vi "main(Test DQMH modules).vi"() -> ()   [LabVIEW 2018, in "Application.lvlib"] (continued)
              tunnel: w10619 -> [w10626 w10656]
              tunnel: [w10637 w10655] -> w10618
              frame False {
                w10623 = T9 {"command"="", "data"=variant} ("element")
                w10636 = T9 {"command"="", "data"=variant} ("element")
                n4774 = To Variant(anything=T3."mux10_1_channel2" ("mux10_1(x6)_encode")) -> (Variant=w10634:variant)
                n4775 = To Variant(anything=T4."demux1_10_channel2" ("demux1_10(x6)_encode")) -> (Variant=w10630:variant)
                n4776 = To Variant(anything=bool[] [FALSE, TRUE, FALSE, FALSE, FALSE, FALSE]) -> (Variant=w10645:variant)
                n4777 = Bundle By Name(cluster=w10636, "command"="MEAS.AllRelaysOFF") -> (w10644:T9)
                n4778 = Bundle By Name(cluster=w10636, "command"="MEAS.mux10-1", "data"=w10634) -> (w10627:T9)
                n4779 = Bundle By Name(cluster=w10636, "command"="MEAS.demux1-10", "data"=w10630) -> (w10628:T9)
                n4780 = Bundle By Name(cluster=w10636, "command"="MEAS.eMIC", "data"=w10645) -> (w10629:T9)
                n4781 = Build Array(w10644, w10627, w10628, w10629) -> (w10622:T9[])
                n4782 = To Variant(anything=w10626) -> (Variant=w10625:variant)
                n4783 = To Variant(anything=w10626) -> (Variant=w10624:variant)
                n4784 = Bundle By Name(cluster=w10623, "command"="MEAS.requestAC", "data"=w10625) -> (w10642:T9)
                n4785 = Bundle By Name(cluster=w10623, "command"="Apps.WaitForEvent", "data"=w10624) -> (w10638:T9)
                n4786 = Bundle By Name(cluster=w10623, "command"="Apps.UI Update 1") -> (w10639:T9)
                n4787 = Bundle By Name(cluster=w10623, "command"="WaitFor") -> (w10621:T9)
                n4788 = Build Array (concatenate)(w10622, w10621, w10642, w10638, w10639) -> (w10637:T9[])
              }
              frame True {
                w10652 = T9 {"command"="", "data"=variant} ("element")
                w10674 = T9 {"command"="", "data"=variant} ("element")
                n4789 = To Variant(anything=T3."mux10_1_channel2" ("mux10_1(x6)_encode")) -> (Variant=w10681:variant)
                n4790 = To Variant(anything=T2."mux6_1_channel2_3" ("mux6_1(3wires)_encode")) -> (Variant=w10679:variant)
                n4791 = To Variant(anything=T4."demux1_10_channel2" ("demux1_10(x6)_encode")) -> (Variant=w10675:variant)
                n4792 = To Variant(anything=bool[] [FALSE, TRUE, FALSE, FALSE, FALSE, FALSE]) -> (Variant=w10671:variant)
                n4793 = Bundle By Name(cluster=w10674, "command"="MEAS.AllRelaysOFF") -> (w10670:T9)
                n4794 = Bundle By Name(cluster=w10674, "command"="MEAS.mux10-1", "data"=w10681) -> (w10669:T9)
                n4795 = Bundle By Name(cluster=w10674, "command"="MEAS.mux6_1", "data"=w10679) -> (w10668:T9)
                n4796 = Bundle By Name(cluster=w10674, "command"="MEAS.demux1-10", "data"=w10675) -> (w10667:T9)
                n4797 = Bundle By Name(cluster=w10674, "command"="MEAS.eMIC", "data"=w10671) -> (w10666:T9)
                n4798 = Build Array(w10670, w10669, w10668, w10667, w10666) -> (w10651:T9[])
                n4799 = To Variant(anything=w10656) -> (Variant=w10654:variant)
                n4800 = To Variant(anything=w10656) -> (Variant=w10653:variant)
                n4801 = Bundle By Name(cluster=w10652, "command"="WaitFor") -> (w10650:T9)
                n4802 = Bundle By Name(cluster=w10652, "command"="MEAS.DMM dual read") -> (w10663:T9)
                n4803 = Bundle By Name(cluster=w10652, "command"="MEAS.requestAC", "data"=w10654) -> (w10662:T9)
                n4804 = Bundle By Name(cluster=w10652, "command"="Apps.WaitForEvent", "data"=w10653) -> (w10657:T9)
                n4805 = Bundle By Name(cluster=w10652, "command"="Apps.UI Update 1") -> (w10658:T9)
                n4806 = Build Array (concatenate)(w10651, w10650, w10663, w10662, w10657, w10658) -> (w10655:T9[])
              }
            }
          }
          frame True {
            n4807 = Bundle By Name(cluster=T9 {"command"="", "data"=variant} ("element"), "command"="Apps.UI Update 1") -> (w10685:T9)
            n4808 = Build Array(w10685) -> (w10684:T9[])
          }
        }
        n4809 = for {
          tunnel: w10600 -> [w10695] mode=indexing
          tunnel: w10608 -> [w10696]
          tunnel: [w10692] -> w10610 mode=indexing
          n4810 = Unbundle By Name(w10695) -> ("command"=w10694:string, "data"=w10693:variant)
          n4811 = call "App enquece.vi"("command data"=w10693, "command"=w10694, "queue in"=w10696) -> ("error out"=w10692:errorcluster)  [unwired: 7 in, 1 out]
        }
        n4812 = Merge Errors(w10611, w10610) -> (w10609:errorcluster)
      }
      frame "Test DRV 9A" {
        w10700 = 9 ("DUT index(0-59)")
        n4813 = disable-structure shown="LOGGING==TRUE" {
          disable-tunnel: w10705 -> [w10788 _]
          frame condition #0 (active) {
            n4814 = Empty String/Path?(string/path=w10788) -> (empty?=w10790:bool)
            n4815 = Select(t="Quece timeout", s=w10790, f=w10788) -> (s? t:f=w10787:string)
            n4816 = call "string log (SubVI).vi"("state Name"=w10787) -> ()  [unwired: 9 in, 2 out]
          }
          frame condition #1 {
          }
        }
        n4817 = Flush Queue(queue=w10706) -> (queue out=w10707:refnum<queue>)  [unwired: 1 in, 2 out]
        n4818 = Decrement(x=w10700) -> (x-1=w10704:i32)
        n4819 = Index Array(array=w10701, index=w10704) -> (element=w10702:refnum<vi>)
        n4820 = call "FGV DRV stand.vi"() -> ("Sub-Test.DCV"=w10697:bool)  [unwired: 10 in, 1 out]
        n4821 = call "FGV Driver Data.vi"("DUT index(1-60)"=w10700) -> ("DUT SC"=w10698:bool)  [unwired: 7 in, 3 out]
        n4822 = property class="ColBox"(reference=w10702, "Value"=u32 10000536 ("DRV 1")) -> ()  [unwired: 1 in, 2 out]
        n4823 = case shown="False" w10698 {
          tunnel: w10700 -> [w10718 _]
          tunnel: [w10717 w10783] -> w10699
          tunnel: w10697 -> [w10716 _]
          frame False {
            n4824 = case shown="True" w10716 {
              tunnel: w10718 -> [w10725 w10755]
              tunnel: [w10736 w10754] -> w10717
              frame False {
                w10722 = T9 {"command"="", "data"=variant} ("element")
                w10735 = T9 {"command"="", "data"=variant} ("element")
                n4825 = To Variant(anything=T3."mux10_1_channel2" ("mux10_1(x6)_encode")) -> (Variant=w10733:variant)
                n4826 = To Variant(anything=T4."demux1_10_channel2" ("demux1_10(x6)_encode")) -> (Variant=w10729:variant)
                n4827 = To Variant(anything=bool[] [FALSE, FALSE, TRUE, FALSE, FALSE, FALSE]) -> (Variant=w10744:variant)
                n4828 = Bundle By Name(cluster=w10735, "command"="MEAS.AllRelaysOFF") -> (w10743:T9)
                n4829 = Bundle By Name(cluster=w10735, "command"="MEAS.mux10-1", "data"=w10733) -> (w10726:T9)
                n4830 = Bundle By Name(cluster=w10735, "command"="MEAS.demux1-10", "data"=w10729) -> (w10727:T9)
                n4831 = Bundle By Name(cluster=w10735, "command"="MEAS.eMIC", "data"=w10744) -> (w10728:T9)
                n4832 = Build Array(w10743, w10726, w10727, w10728) -> (w10721:T9[])
                n4833 = To Variant(anything=w10725) -> (Variant=w10724:variant)
                n4834 = To Variant(anything=w10725) -> (Variant=w10723:variant)
                n4835 = Bundle By Name(cluster=w10722, "command"="MEAS.requestAC", "data"=w10724) -> (w10741:T9)
                n4836 = Bundle By Name(cluster=w10722, "command"="Apps.WaitForEvent", "data"=w10723) -> (w10737:T9)
                n4837 = Bundle By Name(cluster=w10722, "command"="Apps.UI Update 1") -> (w10738:T9)
                n4838 = Bundle By Name(cluster=w10722, "command"="WaitFor") -> (w10720:T9)
                n4839 = Build Array (concatenate)(w10721, w10720, w10741, w10737, w10738) -> (w10736:T9[])
              }
              frame True {
                w10751 = T9 {"command"="", "data"=variant} ("element")
                w10773 = T9 {"command"="", "data"=variant} ("element")
                n4840 = To Variant(anything=T3."mux10_1_channel2" ("mux10_1(x6)_encode")) -> (Variant=w10780:variant)
                n4841 = To Variant(anything=T2."mux6_1_channel3_3" ("mux6_1(3wires)_encode")) -> (Variant=w10778:variant)
                n4842 = To Variant(anything=T4."demux1_10_channel2" ("demux1_10(x6)_encode")) -> (Variant=w10774:variant)
                n4843 = To Variant(anything=bool[] [FALSE, FALSE, TRUE, FALSE, FALSE, FALSE]) -> (Variant=w10770:variant)
                n4844 = Bundle By Name(cluster=w10773, "command"="MEAS.AllRelaysOFF") -> (w10769:T9)
                n4845 = Bundle By Name(cluster=w10773, "command"="MEAS.mux10-1", "data"=w10780) -> (w10768:T9)
                n4846 = Bundle By Name(cluster=w10773, "command"="MEAS.mux6_1", "data"=w10778) -> (w10767:T9)
                n4847 = Bundle By Name(cluster=w10773, "command"="MEAS.demux1-10", "data"=w10774) -> (w10766:T9)
                n4848 = Bundle By Name(cluster=w10773, "command"="MEAS.eMIC", "data"=w10770) -> (w10765:T9)
                n4849 = Build Array(w10769, w10768, w10767, w10766, w10765) -> (w10750:T9[])
                n4850 = To Variant(anything=w10755) -> (Variant=w10753:variant)
                n4851 = To Variant(anything=w10755) -> (Variant=w10752:variant)
                n4852 = Bundle By Name(cluster=w10751, "command"="WaitFor") -> (w10749:T9)
                n4853 = Bundle By Name(cluster=w10751, "command"="MEAS.DMM dual read") -> (w10762:T9)
                n4854 = Bundle By Name(cluster=w10751, "command"="MEAS.requestAC", "data"=w10753) -> (w10761:T9)
                n4855 = Bundle By Name(cluster=w10751, "command"="Apps.WaitForEvent", "data"=w10752) -> (w10756:T9)
                n4856 = Bundle By Name(cluster=w10751, "command"="Apps.UI Update 1") -> (w10757:T9)
                n4857 = Build Array (concatenate)(w10750, w10749, w10762, w10761, w10756, w10757) -> (w10754:T9[])
              }
            }
          }
          frame True {
            n4858 = Bundle By Name(cluster=T9 {"command"="", "data"=variant} ("element"), "command"="Apps.UI Update 1") -> (w10784:T9)
            n4859 = Build Array(w10784) -> (w10783:T9[])
          }
        }
        n4860 = for {
          tunnel: w10699 -> [w10794] mode=indexing
          tunnel: w10707 -> [w10795]
          tunnel: [w10791] -> w10709 mode=indexing
          n4861 = Unbundle By Name(w10794) -> ("command"=w10793:string, "data"=w10792:variant)
          n4862 = call "App enquece.vi"("command data"=w10792, "command"=w10793, "queue in"=w10795) -> ("error out"=w10791:errorcluster)  [unwired: 7 in, 1 out]
        }
        n4863 = Merge Errors(w10710, w10709) -> (w10708:errorcluster)
      }
      frame "Test DRV 10A" {
        w10799 = 10 ("DUT index(0-59)")
        n4864 = disable-structure shown="LOGGING==TRUE" {
          disable-tunnel: w10804 -> [w10887 _]
          frame condition #0 (active) {
            n4865 = Empty String/Path?(string/path=w10887) -> (empty?=w10889:bool)
            n4866 = Select(t="Quece timeout", s=w10889, f=w10887) -> (s? t:f=w10886:string)
            n4867 = call "string log (SubVI).vi"("state Name"=w10886) -> ()  [unwired: 9 in, 2 out]
          }
          frame condition #1 {
          }
        }
        n4868 = Flush Queue(queue=w10805) -> (queue out=w10806:refnum<queue>)  [unwired: 1 in, 2 out]
        n4869 = Decrement(x=w10799) -> (x-1=w10803:i32)
        n4870 = Index Array(array=w10800, index=w10803) -> (element=w10801:refnum<vi>)
        n4871 = call "FGV DRV stand.vi"() -> ("Sub-Test.DCV"=w10796:bool)  [unwired: 10 in, 1 out]
        n4872 = call "FGV Driver Data.vi"("DUT index(1-60)"=w10799) -> ("DUT SC"=w10797:bool)  [unwired: 7 in, 3 out]
        n4873 = property class="ColBox"(reference=w10801, "Value"=u32 10000536 ("DRV 1")) -> ()  [unwired: 1 in, 2 out]
        n4874 = case shown="False" w10797 {
          tunnel: w10799 -> [w10817 _]
          tunnel: [w10816 w10882] -> w10798
          tunnel: w10796 -> [w10815 _]
          frame False {
            n4875 = case shown="False" w10815 {
              tunnel: w10817 -> [w10824 w10854]
              tunnel: [w10835 w10853] -> w10816
              frame False {
                w10821 = T9 {"command"="", "data"=variant} ("element")
                w10834 = T9 {"command"="", "data"=variant} ("element")
                n4876 = To Variant(anything=T3."mux10_1_channel2" ("mux10_1(x6)_encode")) -> (Variant=w10832:variant)
                n4877 = To Variant(anything=T4."demux1_10_channel2" ("demux1_10(x6)_encode")) -> (Variant=w10828:variant)
                n4878 = To Variant(anything=bool[] [FALSE, FALSE, FALSE, TRUE, FALSE, FALSE]) -> (Variant=w10843:variant)
                n4879 = Bundle By Name(cluster=w10834, "command"="MEAS.AllRelaysOFF") -> (w10842:T9)
                n4880 = Bundle By Name(cluster=w10834, "command"="MEAS.mux10-1", "data"=w10832) -> (w10825:T9)
                n4881 = Bundle By Name(cluster=w10834, "command"="MEAS.demux1-10", "data"=w10828) -> (w10826:T9)
                n4882 = Bundle By Name(cluster=w10834, "command"="MEAS.eMIC", "data"=w10843) -> (w10827:T9)
                n4883 = Build Array(w10842, w10825, w10826, w10827) -> (w10820:T9[])
                n4884 = To Variant(anything=w10824) -> (Variant=w10823:variant)
                n4885 = To Variant(anything=w10824) -> (Variant=w10822:variant)
                n4886 = Bundle By Name(cluster=w10821, "command"="MEAS.requestAC", "data"=w10823) -> (w10840:T9)
                n4887 = Bundle By Name(cluster=w10821, "command"="Apps.WaitForEvent", "data"=w10822) -> (w10836:T9)
                n4888 = Bundle By Name(cluster=w10821, "command"="Apps.UI Update 1") -> (w10837:T9)
                n4889 = Bundle By Name(cluster=w10821, "command"="WaitFor") -> (w10819:T9)
                n4890 = Build Array (concatenate)(w10820, w10819, w10840, w10836, w10837) -> (w10835:T9[])
              }
              frame True {
                w10850 = T9 {"command"="", "data"=variant} ("element")
                w10872 = T9 {"command"="", "data"=variant} ("element")
                n4891 = To Variant(anything=T3."mux10_1_channel2" ("mux10_1(x6)_encode")) -> (Variant=w10879:variant)
                n4892 = To Variant(anything=T2."mux6_1_channel4_3" ("mux6_1(3wires)_encode")) -> (Variant=w10877:variant)
                n4893 = To Variant(anything=T4."demux1_10_channel2" ("demux1_10(x6)_encode")) -> (Variant=w10873:variant)
                n4894 = To Variant(anything=bool[] [FALSE, FALSE, FALSE, TRUE, FALSE, FALSE]) -> (Variant=w10869:variant)
                n4895 = Bundle By Name(cluster=w10872, "command"="MEAS.AllRelaysOFF") -> (w10868:T9)
                n4896 = Bundle By Name(cluster=w10872, "command"="MEAS.mux10-1", "data"=w10879) -> (w10867:T9)
                n4897 = Bundle By Name(cluster=w10872, "command"="MEAS.mux6_1", "data"=w10877) -> (w10866:T9)
                n4898 = Bundle By Name(cluster=w10872, "command"="MEAS.demux1-10", "data"=w10873) -> (w10865:T9)
                n4899 = Bundle By Name(cluster=w10872, "command"="MEAS.eMIC", "data"=w10869) -> (w10864:T9)
                n4900 = Build Array(w10868, w10867, w10866, w10865, w10864) -> (w10849:T9[])
                n4901 = To Variant(anything=w10854) -> (Variant=w10852:variant)
                n4902 = To Variant(anything=w10854) -> (Variant=w10851:variant)
                n4903 = Bundle By Name(cluster=w10850, "command"="WaitFor") -> (w10848:T9)
                n4904 = Bundle By Name(cluster=w10850, "command"="MEAS.DMM dual read") -> (w10861:T9)
                n4905 = Bundle By Name(cluster=w10850, "command"="MEAS.requestAC", "data"=w10852) -> (w10860:T9)
                n4906 = Bundle By Name(cluster=w10850, "command"="Apps.WaitForEvent", "data"=w10851) -> (w10855:T9)
                n4907 = Bundle By Name(cluster=w10850, "command"="Apps.UI Update 1") -> (w10856:T9)
                n4908 = Build Array (concatenate)(w10849, w10848, w10861, w10860, w10855, w10856) -> (w10853:T9[])
              }
            }
          }
          frame True {
            n4909 = Bundle By Name(cluster=T9 {"command"="", "data"=variant} ("element"), "command"="Apps.UI Update 1") -> (w10883:T9)
            n4910 = Build Array(w10883) -> (w10882:T9[])
          }
        }
        n4911 = for {
          tunnel: w10798 -> [w10893] mode=indexing
          tunnel: w10806 -> [w10894]
          tunnel: [w10890] -> w10808 mode=indexing
          n4912 = Unbundle By Name(w10893) -> ("command"=w10892:string, "data"=w10891:variant)
          n4913 = call "App enquece.vi"("command data"=w10891, "command"=w10892, "queue in"=w10894) -> ("error out"=w10890:errorcluster)  [unwired: 7 in, 1 out]
        }
        n4914 = Merge Errors(w10809, w10808) -> (w10807:errorcluster)
      }
      frame "Test DRV 11A" {
        w10898 = 11 ("DUT index(0-59)")
        n4915 = disable-structure shown="LOGGING==TRUE" {
          disable-tunnel: w10903 -> [w10986 _]
          frame condition #0 (active) {
            n4916 = Empty String/Path?(string/path=w10986) -> (empty?=w10988:bool)
            n4917 = Select(t="Quece timeout", s=w10988, f=w10986) -> (s? t:f=w10985:string)
            n4918 = call "string log (SubVI).vi"("state Name"=w10985) -> ()  [unwired: 9 in, 2 out]
          }
          frame condition #1 {
          }
        }
        n4919 = Flush Queue(queue=w10904) -> (queue out=w10905:refnum<queue>)  [unwired: 1 in, 2 out]
        n4920 = Decrement(x=w10898) -> (x-1=w10902:i32)
        n4921 = Index Array(array=w10899, index=w10902) -> (element=w10900:refnum<vi>)
        n4922 = call "FGV DRV stand.vi"() -> ("Sub-Test.DCV"=w10895:bool)  [unwired: 10 in, 1 out]
        n4923 = call "FGV Driver Data.vi"("DUT index(1-60)"=w10898) -> ("DUT SC"=w10896:bool)  [unwired: 7 in, 3 out]
        n4924 = property class="ColBox"(reference=w10900, "Value"=u32 10000536 ("DRV 1")) -> ()  [unwired: 1 in, 2 out]
        n4925 = case shown="False" w10896 {
          tunnel: w10898 -> [w10916 _]
          tunnel: [w10915 w10981] -> w10897
          tunnel: w10895 -> [w10914 _]
          frame False {
            n4926 = case shown="True" w10914 {
              tunnel: w10916 -> [w10923 w10953]
              tunnel: [w10934 w10952] -> w10915
              frame False {
                w10920 = T9 {"command"="", "data"=variant} ("element")
                w10933 = T9 {"command"="", "data"=variant} ("element")
                n4927 = To Variant(anything=T3."mux10_1_channel2" ("mux10_1(x6)_encode")) -> (Variant=w10931:variant)
                n4928 = To Variant(anything=T4."demux1_10_channel2" ("demux1_10(x6)_encode")) -> (Variant=w10927:variant)
                n4929 = To Variant(anything=bool[] [FALSE, FALSE, FALSE, FALSE, TRUE, FALSE]) -> (Variant=w10942:variant)
                n4930 = Bundle By Name(cluster=w10933, "command"="MEAS.AllRelaysOFF") -> (w10941:T9)
                n4931 = Bundle By Name(cluster=w10933, "command"="MEAS.mux10-1", "data"=w10931) -> (w10924:T9)
                n4932 = Bundle By Name(cluster=w10933, "command"="MEAS.demux1-10", "data"=w10927) -> (w10925:T9)
                n4933 = Bundle By Name(cluster=w10933, "command"="MEAS.eMIC", "data"=w10942) -> (w10926:T9)
                n4934 = Build Array(w10941, w10924, w10925, w10926) -> (w10919:T9[])
                n4935 = To Variant(anything=w10923) -> (Variant=w10922:variant)
                n4936 = To Variant(anything=w10923) -> (Variant=w10921:variant)
                n4937 = Bundle By Name(cluster=w10920, "command"="MEAS.requestAC", "data"=w10922) -> (w10939:T9)
                n4938 = Bundle By Name(cluster=w10920, "command"="Apps.WaitForEvent", "data"=w10921) -> (w10935:T9)
                n4939 = Bundle By Name(cluster=w10920, "command"="Apps.UI Update 1") -> (w10936:T9)
                n4940 = Bundle By Name(cluster=w10920, "command"="WaitFor") -> (w10918:T9)
                n4941 = Build Array (concatenate)(w10919, w10918, w10939, w10935, w10936) -> (w10934:T9[])
              }
              frame True {
                w10949 = T9 {"command"="", "data"=variant} ("element")
                w10971 = T9 {"command"="", "data"=variant} ("element")
                n4942 = To Variant(anything=T3."mux10_1_channel2" ("mux10_1(x6)_encode")) -> (Variant=w10978:variant)
                n4943 = To Variant(anything=T2."mux6_1_channel5_3" ("mux6_1(3wires)_encode")) -> (Variant=w10976:variant)
                n4944 = To Variant(anything=T4."demux1_10_channel2" ("demux1_10(x6)_encode")) -> (Variant=w10972:variant)
                n4945 = To Variant(anything=bool[] [FALSE, FALSE, FALSE, FALSE, TRUE, FALSE]) -> (Variant=w10968:variant)
                n4946 = Bundle By Name(cluster=w10971, "command"="MEAS.AllRelaysOFF") -> (w10967:T9)
                n4947 = Bundle By Name(cluster=w10971, "command"="MEAS.mux10-1", "data"=w10978) -> (w10966:T9)
                n4948 = Bundle By Name(cluster=w10971, "command"="MEAS.mux6_1", "data"=w10976) -> (w10965:T9)
                n4949 = Bundle By Name(cluster=w10971, "command"="MEAS.demux1-10", "data"=w10972) -> (w10964:T9)
                n4950 = Bundle By Name(cluster=w10971, "command"="MEAS.eMIC", "data"=w10968) -> (w10963:T9)
                n4951 = Build Array(w10967, w10966, w10965, w10964, w10963) -> (w10948:T9[])
                n4952 = To Variant(anything=w10953) -> (Variant=w10951:variant)
                n4953 = To Variant(anything=w10953) -> (Variant=w10950:variant)
                n4954 = Bundle By Name(cluster=w10949, "command"="WaitFor") -> (w10947:T9)
                n4955 = Bundle By Name(cluster=w10949, "command"="MEAS.DMM dual read") -> (w10960:T9)
                n4956 = Bundle By Name(cluster=w10949, "command"="MEAS.requestAC", "data"=w10951) -> (w10959:T9)
                n4957 = Bundle By Name(cluster=w10949, "command"="Apps.WaitForEvent", "data"=w10950) -> (w10954:T9)
                n4958 = Bundle By Name(cluster=w10949, "command"="Apps.UI Update 1") -> (w10955:T9)
                n4959 = Build Array (concatenate)(w10948, w10947, w10960, w10959, w10954, w10955) -> (w10952:T9[])
              }
            }
          }
          frame True {
            n4960 = Bundle By Name(cluster=T9 {"command"="", "data"=variant} ("element"), "command"="Apps.UI Update 1") -> (w10982:T9)
            n4961 = Build Array(w10982) -> (w10981:T9[])
          }
        }
        n4962 = for {
          tunnel: w10897 -> [w10992] mode=indexing
          tunnel: w10905 -> [w10993]
          tunnel: [w10989] -> w10907 mode=indexing
          n4963 = Unbundle By Name(w10992) -> ("command"=w10991:string, "data"=w10990:variant)
          n4964 = call "App enquece.vi"("command data"=w10990, "command"=w10991, "queue in"=w10993) -> ("error out"=w10989:errorcluster)  [unwired: 7 in, 1 out]
        }
        n4965 = Merge Errors(w10908, w10907) -> (w10906:errorcluster)
      }
      frame "Test DRV 12A" {
        w10997 = 12 ("DUT index(0-59)")
        n4966 = disable-structure shown="LOGGING==TRUE" {
          disable-tunnel: w11002 -> [w11085 _]
          frame condition #0 (active) {
            n4967 = Empty String/Path?(string/path=w11085) -> (empty?=w11087:bool)
            n4968 = Select(t="Quece timeout", s=w11087, f=w11085) -> (s? t:f=w11084:string)
            n4969 = call "string log (SubVI).vi"("state Name"=w11084) -> ()  [unwired: 9 in, 2 out]
          }
          frame condition #1 {
          }
        }
        n4970 = Flush Queue(queue=w11003) -> (queue out=w11004:refnum<queue>)  [unwired: 1 in, 2 out]
        n4971 = Decrement(x=w10997) -> (x-1=w11001:i32)
        n4972 = Index Array(array=w10998, index=w11001) -> (element=w10999:refnum<vi>)
        n4973 = call "FGV DRV stand.vi"() -> ("Sub-Test.DCV"=w10994:bool)  [unwired: 10 in, 1 out]
        n4974 = call "FGV Driver Data.vi"("DUT index(1-60)"=w10997) -> ("DUT SC"=w10995:bool)  [unwired: 7 in, 3 out]
        n4975 = property class="ColBox"(reference=w10999, "Value"=u32 10000536 ("DRV 1")) -> ()  [unwired: 1 in, 2 out]
        n4976 = case shown="False" w10995 {
          tunnel: w10997 -> [w11015 _]
          tunnel: [w11014 w11080] -> w10996
          tunnel: w10994 -> [w11013 _]
          frame False {
            n4977 = case shown="True" w11013 {
              tunnel: w11015 -> [w11022 w11052]
              tunnel: [w11033 w11051] -> w11014
              frame False {
                w11019 = T9 {"command"="", "data"=variant} ("element")
                w11032 = T9 {"command"="", "data"=variant} ("element")
                n4978 = To Variant(anything=T3."mux10_1_channel2" ("mux10_1(x6)_encode")) -> (Variant=w11030:variant)
                n4979 = To Variant(anything=T4."demux1_10_channel2" ("demux1_10(x6)_encode")) -> (Variant=w11026:variant)
                n4980 = To Variant(anything=bool[] [FALSE, FALSE, FALSE, FALSE, FALSE, TRUE]) -> (Variant=w11041:variant)
                n4981 = Bundle By Name(cluster=w11032, "command"="MEAS.AllRelaysOFF") -> (w11040:T9)
                n4982 = Bundle By Name(cluster=w11032, "command"="MEAS.mux10-1", "data"=w11030) -> (w11023:T9)
                n4983 = Bundle By Name(cluster=w11032, "command"="MEAS.demux1-10", "data"=w11026) -> (w11024:T9)
                n4984 = Bundle By Name(cluster=w11032, "command"="MEAS.eMIC", "data"=w11041) -> (w11025:T9)
                n4985 = Build Array(w11040, w11023, w11024, w11025) -> (w11018:T9[])
                n4986 = To Variant(anything=w11022) -> (Variant=w11021:variant)
                n4987 = To Variant(anything=w11022) -> (Variant=w11020:variant)
                n4988 = Bundle By Name(cluster=w11019, "command"="MEAS.requestAC", "data"=w11021) -> (w11038:T9)
                n4989 = Bundle By Name(cluster=w11019, "command"="Apps.WaitForEvent", "data"=w11020) -> (w11034:T9)
                n4990 = Bundle By Name(cluster=w11019, "command"="Apps.UI Update 1") -> (w11035:T9)
                n4991 = Bundle By Name(cluster=w11019, "command"="WaitFor") -> (w11017:T9)
                n4992 = Build Array (concatenate)(w11018, w11017, w11038, w11034, w11035) -> (w11033:T9[])
              }
              frame True {
                w11048 = T9 {"command"="", "data"=variant} ("element")
                w11070 = T9 {"command"="", "data"=variant} ("element")
                n4993 = To Variant(anything=T3."mux10_1_channel2" ("mux10_1(x6)_encode")) -> (Variant=w11077:variant)
                n4994 = To Variant(anything=T2."mux6_1_channel6_3" ("mux6_1(3wires)_encode")) -> (Variant=w11075:variant)
                n4995 = To Variant(anything=T4."demux1_10_channel2" ("demux1_10(x6)_encode")) -> (Variant=w11071:variant)
                n4996 = To Variant(anything=bool[] [FALSE, FALSE, FALSE, FALSE, FALSE, TRUE]) -> (Variant=w11067:variant)
                n4997 = Bundle By Name(cluster=w11070, "command"="MEAS.AllRelaysOFF") -> (w11066:T9)
                n4998 = Bundle By Name(cluster=w11070, "command"="MEAS.mux10-1", "data"=w11077) -> (w11065:T9)
                n4999 = Bundle By Name(cluster=w11070, "command"="MEAS.mux6_1", "data"=w11075) -> (w11064:T9)
                n5000 = Bundle By Name(cluster=w11070, "command"="MEAS.demux1-10", "data"=w11071) -> (w11063:T9)
                n5001 = Bundle By Name(cluster=w11070, "command"="MEAS.eMIC", "data"=w11067) -> (w11062:T9)
                n5002 = Build Array(w11066, w11065, w11064, w11063, w11062) -> (w11047:T9[])
                n5003 = To Variant(anything=w11052) -> (Variant=w11050:variant)
                n5004 = To Variant(anything=w11052) -> (Variant=w11049:variant)
                n5005 = Bundle By Name(cluster=w11048, "command"="WaitFor") -> (w11046:T9)
                n5006 = Bundle By Name(cluster=w11048, "command"="MEAS.DMM dual read") -> (w11059:T9)
                n5007 = Bundle By Name(cluster=w11048, "command"="MEAS.requestAC", "data"=w11050) -> (w11058:T9)
                n5008 = Bundle By Name(cluster=w11048, "command"="Apps.WaitForEvent", "data"=w11049) -> (w11053:T9)
                n5009 = Bundle By Name(cluster=w11048, "command"="Apps.UI Update 1") -> (w11054:T9)
                n5010 = Build Array (concatenate)(w11047, w11046, w11059, w11058, w11053, w11054) -> (w11051:T9[])
              }
            }
          }
          frame True {
            n5011 = Bundle By Name(cluster=T9 {"command"="", "data"=variant} ("element"), "command"="Apps.UI Update 1") -> (w11081:T9)
            n5012 = Build Array(w11081) -> (w11080:T9[])
          }
        }
        n5013 = for {
          tunnel: w10996 -> [w11091] mode=indexing
          tunnel: w11004 -> [w11092]
          tunnel: [w11088] -> w11006 mode=indexing
          n5014 = Unbundle By Name(w11091) -> ("command"=w11090:string, "data"=w11089:variant)
          n5015 = call "App enquece.vi"("command data"=w11089, "command"=w11090, "queue in"=w11092) -> ("error out"=w11088:errorcluster)  [unwired: 7 in, 1 out]
        }
        n5016 = Merge Errors(w11007, w11006) -> (w11005:errorcluster)
      }
      frame "Test DRV 13A" {
        w11096 = 13 ("DUT index(0-59)")
        n5017 = disable-structure shown="LOGGING==TRUE" {
          disable-tunnel: w11101 -> [w11184 _]
          frame condition #0 (active) {
            n5018 = Empty String/Path?(string/path=w11184) -> (empty?=w11186:bool)
            n5019 = Select(t="Quece timeout", s=w11186, f=w11184) -> (s? t:f=w11183:string)
            n5020 = call "string log (SubVI).vi"("state Name"=w11183) -> ()  [unwired: 9 in, 2 out]
          }
          frame condition #1 {
          }
        }
        n5021 = Flush Queue(queue=w11102) -> (queue out=w11103:refnum<queue>)  [unwired: 1 in, 2 out]
        n5022 = Decrement(x=w11096) -> (x-1=w11100:i32)
        n5023 = Index Array(array=w11097, index=w11100) -> (element=w11098:refnum<vi>)
        n5024 = call "FGV DRV stand.vi"() -> ("Sub-Test.DCV"=w11093:bool)  [unwired: 10 in, 1 out]
        n5025 = call "FGV Driver Data.vi"("DUT index(1-60)"=w11096) -> ("DUT SC"=w11094:bool)  [unwired: 7 in, 3 out]
        n5026 = property class="ColBox"(reference=w11098, "Value"=u32 10000536 ("DRV 1")) -> ()  [unwired: 1 in, 2 out]
        n5027 = case shown="False" w11094 {
          tunnel: w11096 -> [w11114 _]
          tunnel: [w11113 w11179] -> w11095
          tunnel: w11093 -> [w11112 _]
          frame False {
            n5028 = case shown="False" w11112 {
              tunnel: w11114 -> [w11121 w11151]
              tunnel: [w11132 w11150] -> w11113
              frame False {
                w11118 = T9 {"command"="", "data"=variant} ("element")
                w11131 = T9 {"command"="", "data"=variant} ("element")
                n5029 = To Variant(anything=T3."mux10_1_channel3" ("mux10_1(x6)_encode")) -> (Variant=w11129:variant)
                n5030 = To Variant(anything=T4."demux1_10_channel3" ("demux1_10(x6)_encode")) -> (Variant=w11125:variant)
                n5031 = To Variant(anything=bool[] [TRUE, FALSE, FALSE, FALSE, FALSE, FALSE]) -> (Variant=w11140:variant)
                n5032 = Bundle By Name(cluster=w11131, "command"="MEAS.AllRelaysOFF") -> (w11139:T9)
                n5033 = Bundle By Name(cluster=w11131, "command"="MEAS.mux10-1", "data"=w11129) -> (w11122:T9)
                n5034 = Bundle By Name(cluster=w11131, "command"="MEAS.demux1-10", "data"=w11125) -> (w11123:T9)
                n5035 = Bundle By Name(cluster=w11131, "command"="MEAS.eMIC", "data"=w11140) -> (w11124:T9)
                n5036 = Build Array(w11139, w11122, w11123, w11124) -> (w11117:T9[])
                n5037 = To Variant(anything=w11121) -> (Variant=w11120:variant)
                n5038 = To Variant(anything=w11121) -> (Variant=w11119:variant)
                n5039 = Bundle By Name(cluster=w11118, "command"="MEAS.requestAC", "data"=w11120) -> (w11137:T9)
                n5040 = Bundle By Name(cluster=w11118, "command"="Apps.WaitForEvent", "data"=w11119) -> (w11133:T9)
                n5041 = Bundle By Name(cluster=w11118, "command"="Apps.UI Update 1") -> (w11134:T9)
                n5042 = Bundle By Name(cluster=w11118, "command"="WaitFor") -> (w11116:T9)
                n5043 = Build Array (concatenate)(w11117, w11116, w11137, w11133, w11134) -> (w11132:T9[])
              }
              frame True {
                w11147 = T9 {"command"="", "data"=variant} ("element")
                w11169 = T9 {"command"="", "data"=variant} ("element")
                n5044 = To Variant(anything=T3."mux10_1_channel3" ("mux10_1(x6)_encode")) -> (Variant=w11176:variant)
                n5045 = To Variant(anything=T2."mux6_1_channel1_3" ("mux6_1(3wires)_encode")) -> (Variant=w11174:variant)
                n5046 = To Variant(anything=T4."demux1_10_channel3" ("demux1_10(x6)_encode")) -> (Variant=w11170:variant)
                n5047 = To Variant(anything=bool[] [TRUE, FALSE, FALSE, FALSE, FALSE, FALSE]) -> (Variant=w11166:variant)
                n5048 = Bundle By Name(cluster=w11169, "command"="MEAS.AllRelaysOFF") -> (w11165:T9)
                n5049 = Bundle By Name(cluster=w11169, "command"="MEAS.mux10-1", "data"=w11176) -> (w11164:T9)
                n5050 = Bundle By Name(cluster=w11169, "command"="MEAS.mux6_1", "data"=w11174) -> (w11163:T9)
                n5051 = Bundle By Name(cluster=w11169, "command"="MEAS.demux1-10", "data"=w11170) -> (w11162:T9)
                n5052 = Bundle By Name(cluster=w11169, "command"="MEAS.eMIC", "data"=w11166) -> (w11161:T9)
                n5053 = Build Array(w11165, w11164, w11163, w11162, w11161) -> (w11146:T9[])
                n5054 = To Variant(anything=w11151) -> (Variant=w11149:variant)
                n5055 = To Variant(anything=w11151) -> (Variant=w11148:variant)
                n5056 = Bundle By Name(cluster=w11147, "command"="WaitFor") -> (w11145:T9)
                n5057 = Bundle By Name(cluster=w11147, "command"="MEAS.DMM dual read") -> (w11158:T9)
                n5058 = Bundle By Name(cluster=w11147, "command"="MEAS.requestAC", "data"=w11149) -> (w11157:T9)
                n5059 = Bundle By Name(cluster=w11147, "command"="Apps.WaitForEvent", "data"=w11148) -> (w11152:T9)
                n5060 = Bundle By Name(cluster=w11147, "command"="Apps.UI Update 1") -> (w11153:T9)
                n5061 = Build Array (concatenate)(w11146, w11145, w11158, w11157, w11152, w11153) -> (w11150:T9[])
              }
            }
          }
          frame True {
            n5062 = Bundle By Name(cluster=T9 {"command"="", "data"=variant} ("element"), "command"="Apps.UI Update 1") -> (w11180:T9)
            n5063 = Build Array(w11180) -> (w11179:T9[])
          }
        }
        n5064 = for {
          tunnel: w11095 -> [w11190] mode=indexing
          tunnel: w11103 -> [w11191]
          tunnel: [w11187] -> w11105 mode=indexing
          n5065 = Unbundle By Name(w11190) -> ("command"=w11189:string, "data"=w11188:variant)
          n5066 = call "App enquece.vi"("command data"=w11188, "command"=w11189, "queue in"=w11191) -> ("error out"=w11187:errorcluster)  [unwired: 7 in, 1 out]
        }
        n5067 = Merge Errors(w11106, w11105) -> (w11104:errorcluster)
      }
      frame "Test DRV 14A" {
        w11195 = 14 ("DUT index(0-59)")
        n5068 = disable-structure shown="LOGGING==TRUE" {
          disable-tunnel: w11200 -> [w11283 _]
          frame condition #0 (active) {
            n5069 = Empty String/Path?(string/path=w11283) -> (empty?=w11285:bool)
            n5070 = Select(t="Quece timeout", s=w11285, f=w11283) -> (s? t:f=w11282:string)
            n5071 = call "string log (SubVI).vi"("state Name"=w11282) -> ()  [unwired: 9 in, 2 out]
          }
          frame condition #1 {
          }
        }
        n5072 = Flush Queue(queue=w11201) -> (queue out=w11202:refnum<queue>)  [unwired: 1 in, 2 out]
        n5073 = Decrement(x=w11195) -> (x-1=w11199:i32)
        n5074 = Index Array(array=w11196, index=w11199) -> (element=w11197:refnum<vi>)
        n5075 = call "FGV DRV stand.vi"() -> ("Sub-Test.DCV"=w11192:bool)  [unwired: 10 in, 1 out]
        n5076 = call "FGV Driver Data.vi"("DUT index(1-60)"=w11195) -> ("DUT SC"=w11193:bool)  [unwired: 7 in, 3 out]
        n5077 = property class="ColBox"(reference=w11197, "Value"=u32 10000536 ("DRV 1")) -> ()  [unwired: 1 in, 2 out]
        n5078 = case shown="False" w11193 {
          tunnel: w11195 -> [w11213 _]
          tunnel: [w11212 w11278] -> w11194
          tunnel: w11192 -> [w11211 _]
          frame False {
            n5079 = case shown="True" w11211 {
              tunnel: w11213 -> [w11220 w11250]
              tunnel: [w11231 w11249] -> w11212
              frame False {
                w11217 = T9 {"command"="", "data"=variant} ("element")
                w11230 = T9 {"command"="", "data"=variant} ("element")
                n5080 = To Variant(anything=T3."mux10_1_channel3" ("mux10_1(x6)_encode")) -> (Variant=w11228:variant)
                n5081 = To Variant(anything=T4."demux1_10_channel3" ("demux1_10(x6)_encode")) -> (Variant=w11224:variant)
                n5082 = To Variant(anything=bool[] [FALSE, TRUE, FALSE, FALSE, FALSE, FALSE]) -> (Variant=w11239:variant)
                n5083 = Bundle By Name(cluster=w11230, "command"="MEAS.AllRelaysOFF") -> (w11238:T9)
                n5084 = Bundle By Name(cluster=w11230, "command"="MEAS.mux10-1", "data"=w11228) -> (w11221:T9)
                n5085 = Bundle By Name(cluster=w11230, "command"="MEAS.demux1-10", "data"=w11224) -> (w11222:T9)
                n5086 = Bundle By Name(cluster=w11230, "command"="MEAS.eMIC", "data"=w11239) -> (w11223:T9)
                n5087 = Build Array(w11238, w11221, w11222, w11223) -> (w11216:T9[])
                n5088 = To Variant(anything=w11220) -> (Variant=w11219:variant)
                n5089 = To Variant(anything=w11220) -> (Variant=w11218:variant)
                n5090 = Bundle By Name(cluster=w11217, "command"="MEAS.requestAC", "data"=w11219) -> (w11236:T9)
                n5091 = Bundle By Name(cluster=w11217, "command"="Apps.WaitForEvent", "data"=w11218) -> (w11232:T9)
                n5092 = Bundle By Name(cluster=w11217, "command"="Apps.UI Update 1") -> (w11233:T9)
                n5093 = Bundle By Name(cluster=w11217, "command"="WaitFor") -> (w11215:T9)
                n5094 = Build Array (concatenate)(w11216, w11215, w11236, w11232, w11233) -> (w11231:T9[])
              }
              frame True {
                w11246 = T9 {"command"="", "data"=variant} ("element")
                w11268 = T9 {"command"="", "data"=variant} ("element")
                n5095 = To Variant(anything=T3."mux10_1_channel3" ("mux10_1(x6)_encode")) -> (Variant=w11275:variant)
                n5096 = To Variant(anything=T2."mux6_1_channel2_3" ("mux6_1(3wires)_encode")) -> (Variant=w11273:variant)
                n5097 = To Variant(anything=T4."demux1_10_channel3" ("demux1_10(x6)_encode")) -> (Variant=w11269:variant)
                n5098 = To Variant(anything=bool[] [FALSE, TRUE, FALSE, FALSE, FALSE, FALSE]) -> (Variant=w11265:variant)
                n5099 = Bundle By Name(cluster=w11268, "command"="MEAS.AllRelaysOFF") -> (w11264:T9)
                n5100 = Bundle By Name(cluster=w11268, "command"="MEAS.mux10-1", "data"=w11275) -> (w11263:T9)
                n5101 = Bundle By Name(cluster=w11268, "command"="MEAS.mux6_1", "data"=w11273) -> (w11262:T9)
                n5102 = Bundle By Name(cluster=w11268, "command"="MEAS.demux1-10", "data"=w11269) -> (w11261:T9)
                n5103 = Bundle By Name(cluster=w11268, "command"="MEAS.eMIC", "data"=w11265) -> (w11260:T9)
                n5104 = Build Array(w11264, w11263, w11262, w11261, w11260) -> (w11245:T9[])
                n5105 = To Variant(anything=w11250) -> (Variant=w11248:variant)
                n5106 = To Variant(anything=w11250) -> (Variant=w11247:variant)
                n5107 = Bundle By Name(cluster=w11246, "command"="WaitFor") -> (w11244:T9)
                n5108 = Bundle By Name(cluster=w11246, "command"="MEAS.DMM dual read") -> (w11257:T9)
                n5109 = Bundle By Name(cluster=w11246, "command"="MEAS.requestAC", "data"=w11248) -> (w11256:T9)
                n5110 = Bundle By Name(cluster=w11246, "command"="Apps.WaitForEvent", "data"=w11247) -> (w11251:T9)
                n5111 = Bundle By Name(cluster=w11246, "command"="Apps.UI Update 1") -> (w11252:T9)
                n5112 = Build Array (concatenate)(w11245, w11244, w11257, w11256, w11251, w11252) -> (w11249:T9[])
              }
            }
          }
          frame True {
            n5113 = Bundle By Name(cluster=T9 {"command"="", "data"=variant} ("element"), "command"="Apps.UI Update 1") -> (w11279:T9)
            n5114 = Build Array(w11279) -> (w11278:T9[])
          }
        }
        n5115 = for {
          tunnel: w11194 -> [w11289] mode=indexing
          tunnel: w11202 -> [w11290]
          tunnel: [w11286] -> w11204 mode=indexing
          n5116 = Unbundle By Name(w11289) -> ("command"=w11288:string, "data"=w11287:variant)
          n5117 = call "App enquece.vi"("command data"=w11287, "command"=w11288, "queue in"=w11290) -> ("error out"=w11286:errorcluster)  [unwired: 7 in, 1 out]
        }
        n5118 = Merge Errors(w11205, w11204) -> (w11203:errorcluster)
      }
      frame "Test DRV 15A" {
        w11294 = 15 ("DUT index(0-59)")
        n5119 = disable-structure shown="LOGGING==TRUE" {
          disable-tunnel: w11299 -> [w11382 _]
          frame condition #0 (active) {
            n5120 = Empty String/Path?(string/path=w11382) -> (empty?=w11384:bool)
            n5121 = Select(t="Quece timeout", s=w11384, f=w11382) -> (s? t:f=w11381:string)
            n5122 = call "string log (SubVI).vi"("state Name"=w11381) -> ()  [unwired: 9 in, 2 out]
          }
          frame condition #1 {
          }
        }
        n5123 = Flush Queue(queue=w11300) -> (queue out=w11301:refnum<queue>)  [unwired: 1 in, 2 out]
        n5124 = Decrement(x=w11294) -> (x-1=w11298:i32)
        n5125 = Index Array(array=w11295, index=w11298) -> (element=w11296:refnum<vi>)
        n5126 = call "FGV DRV stand.vi"() -> ("Sub-Test.DCV"=w11291:bool)  [unwired: 10 in, 1 out]
        n5127 = call "FGV Driver Data.vi"("DUT index(1-60)"=w11294) -> ("DUT SC"=w11292:bool)  [unwired: 7 in, 3 out]
        n5128 = property class="ColBox"(reference=w11296, "Value"=u32 10000536 ("DRV 1")) -> ()  [unwired: 1 in, 2 out]
        n5129 = case shown="False" w11292 {
          tunnel: w11294 -> [w11312 _]
          tunnel: [w11311 w11377] -> w11293
          tunnel: w11291 -> [w11310 _]
          frame False {
            n5130 = case shown="True" w11310 {
              tunnel: w11312 -> [w11319 w11349]
              tunnel: [w11330 w11348] -> w11311
              frame False {
                w11316 = T9 {"command"="", "data"=variant} ("element")
                w11329 = T9 {"command"="", "data"=variant} ("element")
                n5131 = To Variant(anything=T3."mux10_1_channel3" ("mux10_1(x6)_encode")) -> (Variant=w11327:variant)
                n5132 = To Variant(anything=T4."demux1_10_channel3" ("demux1_10(x6)_encode")) -> (Variant=w11323:variant)
                n5133 = To Variant(anything=bool[] [FALSE, FALSE, TRUE, FALSE, FALSE, FALSE]) -> (Variant=w11338:variant)
                n5134 = Bundle By Name(cluster=w11329, "command"="MEAS.AllRelaysOFF") -> (w11337:T9)
                n5135 = Bundle By Name(cluster=w11329, "command"="MEAS.mux10-1", "data"=w11327) -> (w11320:T9)
                n5136 = Bundle By Name(cluster=w11329, "command"="MEAS.demux1-10", "data"=w11323) -> (w11321:T9)
                n5137 = Bundle By Name(cluster=w11329, "command"="MEAS.eMIC", "data"=w11338) -> (w11322:T9)
                n5138 = Build Array(w11337, w11320, w11321, w11322) -> (w11315:T9[])
                n5139 = To Variant(anything=w11319) -> (Variant=w11318:variant)
                n5140 = To Variant(anything=w11319) -> (Variant=w11317:variant)
                n5141 = Bundle By Name(cluster=w11316, "command"="MEAS.requestAC", "data"=w11318) -> (w11335:T9)
                n5142 = Bundle By Name(cluster=w11316, "command"="Apps.WaitForEvent", "data"=w11317) -> (w11331:T9)
                n5143 = Bundle By Name(cluster=w11316, "command"="Apps.UI Update 1") -> (w11332:T9)
                n5144 = Bundle By Name(cluster=w11316, "command"="WaitFor") -> (w11314:T9)
                n5145 = Build Array (concatenate)(w11315, w11314, w11335, w11331, w11332) -> (w11330:T9[])
              }
              frame True {
                w11345 = T9 {"command"="", "data"=variant} ("element")
                w11367 = T9 {"command"="", "data"=variant} ("element")
                n5146 = To Variant(anything=T3."mux10_1_channel3" ("mux10_1(x6)_encode")) -> (Variant=w11374:variant)
                n5147 = To Variant(anything=T2."mux6_1_channel3_3" ("mux6_1(3wires)_encode")) -> (Variant=w11372:variant)
                n5148 = To Variant(anything=T4."demux1_10_channel3" ("demux1_10(x6)_encode")) -> (Variant=w11368:variant)
                n5149 = To Variant(anything=bool[] [FALSE, FALSE, TRUE, FALSE, FALSE, FALSE]) -> (Variant=w11364:variant)
                n5150 = Bundle By Name(cluster=w11367, "command"="MEAS.AllRelaysOFF") -> (w11363:T9)
                n5151 = Bundle By Name(cluster=w11367, "command"="MEAS.mux10-1", "data"=w11374) -> (w11362:T9)
                n5152 = Bundle By Name(cluster=w11367, "command"="MEAS.mux6_1", "data"=w11372) -> (w11361:T9)
                n5153 = Bundle By Name(cluster=w11367, "command"="MEAS.demux1-10", "data"=w11368) -> (w11360:T9)
                n5154 = Bundle By Name(cluster=w11367, "command"="MEAS.eMIC", "data"=w11364) -> (w11359:T9)
                n5155 = Build Array(w11363, w11362, w11361, w11360, w11359) -> (w11344:T9[])
                n5156 = To Variant(anything=w11349) -> (Variant=w11347:variant)
                n5157 = To Variant(anything=w11349) -> (Variant=w11346:variant)
                n5158 = Bundle By Name(cluster=w11345, "command"="WaitFor") -> (w11343:T9)
                n5159 = Bundle By Name(cluster=w11345, "command"="MEAS.DMM dual read") -> (w11356:T9)
                n5160 = Bundle By Name(cluster=w11345, "command"="MEAS.requestAC", "data"=w11347) -> (w11355:T9)
                n5161 = Bundle By Name(cluster=w11345, "command"="Apps.WaitForEvent", "data"=w11346) -> (w11350:T9)
                n5162 = Bundle By Name(cluster=w11345, "command"="Apps.UI Update 1") -> (w11351:T9)
                n5163 = Build Array (concatenate)(w11344, w11343, w11356, w11355, w11350, w11351) -> (w11348:T9[])
              }
            }
          }
          frame True {
            n5164 = Bundle By Name(cluster=T9 {"command"="", "data"=variant} ("element"), "command"="Apps.UI Update 1") -> (w11378:T9)
            n5165 = Build Array(w11378) -> (w11377:T9[])
          }
        }
        n5166 = for {
          tunnel: w11293 -> [w11388] mode=indexing
          tunnel: w11301 -> [w11389]
          tunnel: [w11385] -> w11303 mode=indexing
          n5167 = Unbundle By Name(w11388) -> ("command"=w11387:string, "data"=w11386:variant)
          n5168 = call "App enquece.vi"("command data"=w11386, "command"=w11387, "queue in"=w11389) -> ("error out"=w11385:errorcluster)  [unwired: 7 in, 1 out]
        }
        n5169 = Merge Errors(w11304, w11303) -> (w11302:errorcluster)
      }
      frame "Test DRV 16A" {
        w11393 = 16 ("DUT index(0-59)")
        n5170 = disable-structure shown="LOGGING==TRUE" {
          disable-tunnel: w11398 -> [w11481 _]
          frame condition #0 (active) {
            n5171 = Empty String/Path?(string/path=w11481) -> (empty?=w11483:bool)
            n5172 = Select(t="Quece timeout", s=w11483, f=w11481) -> (s? t:f=w11480:string)
            n5173 = call "string log (SubVI).vi"("state Name"=w11480) -> ()  [unwired: 9 in, 2 out]
          }
          frame condition #1 {
          }
        }
        n5174 = Flush Queue(queue=w11399) -> (queue out=w11400:refnum<queue>)  [unwired: 1 in, 2 out]
        n5175 = Decrement(x=w11393) -> (x-1=w11397:i32)
        n5176 = Index Array(array=w11394, index=w11397) -> (element=w11395:refnum<vi>)
        n5177 = call "FGV DRV stand.vi"() -> ("Sub-Test.DCV"=w11390:bool)  [unwired: 10 in, 1 out]
        n5178 = call "FGV Driver Data.vi"("DUT index(1-60)"=w11393) -> ("DUT SC"=w11391:bool)  [unwired: 7 in, 3 out]
        n5179 = property class="ColBox"(reference=w11395, "Value"=u32 10000536 ("DRV 1")) -> ()  [unwired: 1 in, 2 out]
        n5180 = case shown="False" w11391 {
          tunnel: w11393 -> [w11411 _]
          tunnel: [w11410 w11476] -> w11392
          tunnel: w11390 -> [w11409 _]
          frame False {
            n5181 = case shown="False" w11409 {
              tunnel: w11411 -> [w11418 w11448]
              tunnel: [w11429 w11447] -> w11410
              frame False {
                w11415 = T9 {"command"="", "data"=variant} ("element")
                w11428 = T9 {"command"="", "data"=variant} ("element")
                n5182 = To Variant(anything=T3."mux10_1_channel3" ("mux10_1(x6)_encode")) -> (Variant=w11426:variant)
                n5183 = To Variant(anything=T4."demux1_10_channel3" ("demux1_10(x6)_encode")) -> (Variant=w11422:variant)
                n5184 = To Variant(anything=bool[] [FALSE, FALSE, FALSE, TRUE, FALSE, FALSE]) -> (Variant=w11437:variant)
                n5185 = Bundle By Name(cluster=w11428, "command"="MEAS.AllRelaysOFF") -> (w11436:T9)
                n5186 = Bundle By Name(cluster=w11428, "command"="MEAS.mux10-1", "data"=w11426) -> (w11419:T9)
                n5187 = Bundle By Name(cluster=w11428, "command"="MEAS.demux1-10", "data"=w11422) -> (w11420:T9)
                n5188 = Bundle By Name(cluster=w11428, "command"="MEAS.eMIC", "data"=w11437) -> (w11421:T9)
                n5189 = Build Array(w11436, w11419, w11420, w11421) -> (w11414:T9[])
                n5190 = To Variant(anything=w11418) -> (Variant=w11417:variant)
                n5191 = To Variant(anything=w11418) -> (Variant=w11416:variant)
                n5192 = Bundle By Name(cluster=w11415, "command"="MEAS.requestAC", "data"=w11417) -> (w11434:T9)
                n5193 = Bundle By Name(cluster=w11415, "command"="Apps.WaitForEvent", "data"=w11416) -> (w11430:T9)
                n5194 = Bundle By Name(cluster=w11415, "command"="Apps.UI Update 1") -> (w11431:T9)
                n5195 = Bundle By Name(cluster=w11415, "command"="WaitFor") -> (w11413:T9)
                n5196 = Build Array (concatenate)(w11414, w11413, w11434, w11430, w11431) -> (w11429:T9[])
              }
              frame True {
                w11444 = T9 {"command"="", "data"=variant} ("element")
                w11466 = T9 {"command"="", "data"=variant} ("element")
                n5197 = To Variant(anything=T3."mux10_1_channel3" ("mux10_1(x6)_encode")) -> (Variant=w11473:variant)
                n5198 = To Variant(anything=T2."mux6_1_channel4_3" ("mux6_1(3wires)_encode")) -> (Variant=w11471:variant)
                n5199 = To Variant(anything=T4."demux1_10_channel3" ("demux1_10(x6)_encode")) -> (Variant=w11467:variant)
                n5200 = To Variant(anything=bool[] [FALSE, FALSE, FALSE, TRUE, FALSE, FALSE]) -> (Variant=w11463:variant)
                n5201 = Bundle By Name(cluster=w11466, "command"="MEAS.AllRelaysOFF") -> (w11462:T9)
                n5202 = Bundle By Name(cluster=w11466, "command"="MEAS.mux10-1", "data"=w11473) -> (w11461:T9)
                n5203 = Bundle By Name(cluster=w11466, "command"="MEAS.mux6_1", "data"=w11471) -> (w11460:T9)
                n5204 = Bundle By Name(cluster=w11466, "command"="MEAS.demux1-10", "data"=w11467) -> (w11459:T9)
                n5205 = Bundle By Name(cluster=w11466, "command"="MEAS.eMIC", "data"=w11463) -> (w11458:T9)
                n5206 = Build Array(w11462, w11461, w11460, w11459, w11458) -> (w11443:T9[])
                n5207 = To Variant(anything=w11448) -> (Variant=w11446:variant)
                n5208 = To Variant(anything=w11448) -> (Variant=w11445:variant)
                n5209 = Bundle By Name(cluster=w11444, "command"="WaitFor") -> (w11442:T9)
                n5210 = Bundle By Name(cluster=w11444, "command"="MEAS.DMM dual read") -> (w11455:T9)
                n5211 = Bundle By Name(cluster=w11444, "command"="MEAS.requestAC", "data"=w11446) -> (w11454:T9)
                n5212 = Bundle By Name(cluster=w11444, "command"="Apps.WaitForEvent", "data"=w11445) -> (w11449:T9)
                n5213 = Bundle By Name(cluster=w11444, "command"="Apps.UI Update 1") -> (w11450:T9)
                n5214 = Build Array (concatenate)(w11443, w11442, w11455, w11454, w11449, w11450) -> (w11447:T9[])
              }
            }
          }
          frame True {
            n5215 = Bundle By Name(cluster=T9 {"command"="", "data"=variant} ("element"), "command"="Apps.UI Update 1") -> (w11477:T9)
            n5216 = Build Array(w11477) -> (w11476:T9[])
